vi "ChangeArrayInWindow(SubVI).vi"(6 "CmbBox Refnum":refnum<vi>, 7 "Digital in":refnum<vi>, 8 "Error In":errorcluster, 9 "Arr Refnum":refnum<vi>, 10 "Clust Refnum":refnum<vi>, 11 "Enum in":refnum<vi>) -> (0 "Error Out":errorcluster)   [LabVIEW 2018]
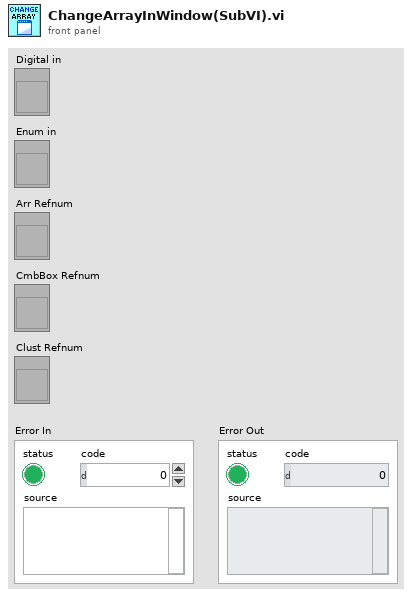
[diagram p1: front panel]
types:
  T1 = typedef "Line.ctl" = cluster{"Width":dbl, "Color":i64, "Array Oy":dbl[], "Array Ox":dbl[], "Name":string, "Plot Visible":T2}
  T2 = typedef "View.ctl" = bool
  T3 = typedef "LVComboBoxStrsAndValuesArrayTypeDef.ctl" = cluster{"String":string, "Value":string}[]
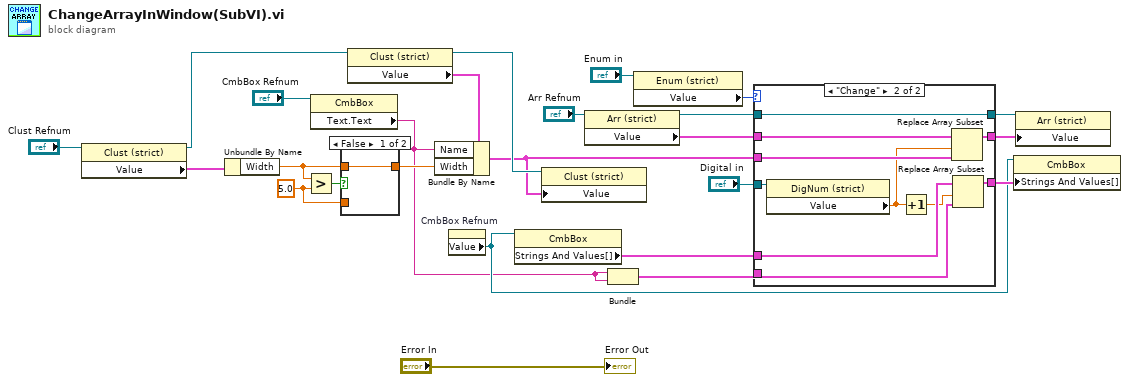
[diagram p0: block diagram]
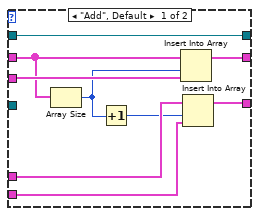
[diagram p2: hidden frame]
diagram:
  w11 = 5.0 ("y")
  n1 = property on="Property Node" class="Clust (strict)"(reference="Clust Refnum") -> (reference out=w18:refnum<vi>, "Value"=w17:T1)  [unwired: 1 in, 1 out]
  n2 = Unbundle By Name(w17) -> ("Width"=w10:dbl)
  n3 = Greater?(x=w10, y=w11) -> (0:w12:bool)
  n4 = property on="Property Node" class="CmbBox"(reference="CmbBox Refnum") -> ("Text.Text"=w1:string)  [unwired: 1 in, 2 out]
  n5 = case shown="False" w12 {
    tunnel: w11 -> [_ w27]
    tunnel: w10 -> [w26 _]
    tunnel: [w26 w27] -> w2
    frame False {
    }
    frame True {
    }
  }
  n6 = property on="Property Node" class="Clust (strict)"(reference=w18) -> (reference out=w20:refnum<vi>, "Value"=w15:T1)  [unwired: 1 in, 1 out]
  n7 = Bundle By Name(cluster=w15, "Name"=w1, "Width"=w2) -> (w9:T1)
  n8 = property on="CmbBox Refnum" class="LVObjRef (strict)"() -> ("Value"=w4:refnum<vi>)  [unwired: 2 in, 2 out]
  n9 = property on="Property Node" class="CmbBox"(reference=w4) -> ("Strings And Values[]"=w8:T3)  [unwired: 1 in, 2 out]
  n10 = property on="Property Node" class="Clust (strict)"(reference=w20, "Value"=w9) -> ()  [unwired: 1 in, 2 out]
  n11 = property on="Property Node" class="Arr (strict)"(reference="Arr Refnum") -> (reference out=w21:refnum<vi>, "Value"=w14:T1[])  [unwired: 1 in, 1 out]
  n12 = Bundle("Text.Text"=w1, "Text.Text"=w1) -> (w13:cluster{"Text.Text":string, "Text.Text":string})  [unwired: 1 in]
  n13 = property on="Property Node" class="Enum (strict)"(reference="Enum in") -> ("Value"=w25:enum16{"Add", "Change"})  [unwired: 1 in, 2 out]
  n14 = case shown="\"Change\"" w25 {
    tunnel: w8 -> [w34 w46]
    tunnel: w9 -> [w36 w45]
    tunnel: w13 -> [w33 w44]
    tunnel: w14 -> [w30 w43]
    tunnel: w21 -> [w31 w40]
    tunnel: [w35 w42] -> w22
    tunnel: [w32 w41] -> w23
    tunnel: [w31 w40] -> w24
    tunnel: "Digital in" -> [_ w39]
    frame "Add", Default {
      n15 = Array Size(array=w30) -> (size(s)=w29:i32)
      n16 = Increment(x=w29) -> (x+1=w28:i32)
      n17 = Insert Into Array(array=w30, index=w29, new element=w36) -> (w35:T1[])
      n18 = Insert Into Array(array=w34, index=w28, new element=w33) -> (w32:T3)
    }
    frame "Change" {
      n19 = property on="Property Node" class="DigNum (strict)"(reference=w39) -> ("Value"=w38:dbl)  [unwired: 1 in, 2 out]
      n20 = Increment(x=w38) -> (x+1=w37:dbl)
      n21 = Replace Array Subset(array=w43, new element=w45, index=w38) -> (w42:T1[])
      n22 = Replace Array Subset(array=w46, new element=w44, index=w37) -> (w41:T3)
    }
  }
  n23 = property on="Property Node" class="CmbBox"(reference=w4, "Strings And Values[]"=w23) -> ()  [unwired: 1 in, 2 out]
  n24 = property on="Property Node" class="Arr (strict)"(reference=w24, "Value"=w22) -> ()  [unwired: 1 in, 2 out]
  "Error Out" <- "Error In"
